vi "Find Album.vi"(8 "error in (no error)":errorcluster, 9 "Artist":string, 10 "Album":string, 11 "MusicLibrary in":refnum<class "MusicLibrary.lvclass">) -> (0 "error out":errorcluster, 2 "Album":refnum<class "Album.lvclass">, 3 "MusicLibrary out":refnum<class "MusicLibrary.lvclass">, 5 "Found?":bool)   [LabVIEW 2015, in "MusicLibrary.lvclass"]
uses:
  MusicLibrary.lvclass
  Album/Album.lvclass
  MusicElementLibrary.lvclass/MusicElementLibrary.ctl
  MusicElement.lvclass/MusicElement.ctl
  Album/Album.lvclass/Album.ctl
  MusicElement.lvclass
  MusicElementLibrary.lvclass
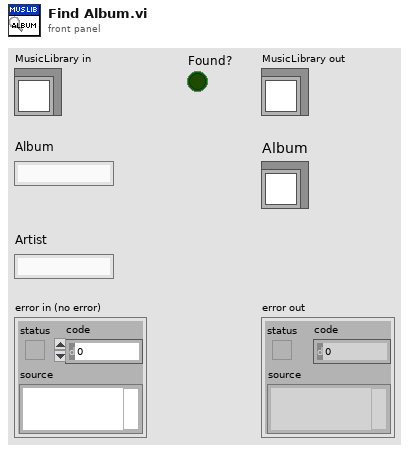
[diagram p1: front panel]
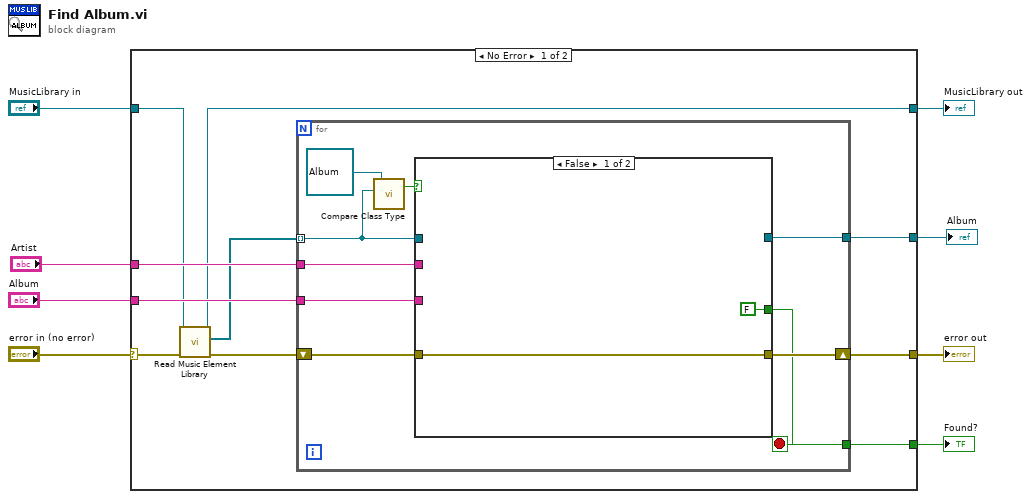
[diagram p0: block diagram]
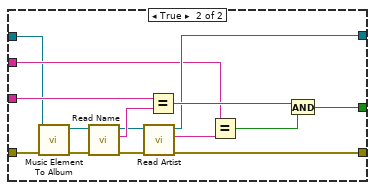
[diagram p2: hidden frame]
diagram:
  n1 = case shown="No Error" "error in (no error)" {
    selector: "error in (no error)" -> [w13 w46]
    tunnel: [w17 w46] -> w7
    tunnel: [w10 w45] -> w5
    tunnel: "MusicLibrary in" -> [w11 w45]
    tunnel: "Album" -> [w18 _]
    tunnel: [w15 _] -> w2
    tunnel: [w16 _] -> w3
    tunnel: "Artist" -> [w14 _]
    frame No Error {
      n2 = call "Read Music Element Library.vi"("error in (no error)"=w13, "MusicElementLibrary in"=w11) -> ("error out"=w12:errorcluster, "Music Element Library"=w9:refnum<class "MusicElement.lvclass">[], "MusicElementLibrary out"=w10:refnum<class "MusicLibrary.lvclass">)  [unwired: 7 in]
      n3 = for {
        tunnel: w9 -> [w19] mode=indexing
        shift-right: [w26] -> w17
        shift-left: w12 -> [w21]
        tunnel: w18 -> [w27]
        tunnel: [w25] -> w16
        tunnel: [w24] -> w15
        tunnel: w14 -> [w23]
        stop <- w25 stop-if-true
        n4 = call "Compare Class Type.vi"("MusicElement Check"=w19, "MusicElement in"=refnum<class "Album.lvclass"> refnum ("Album")) -> ("Same Class Type?"=w22:bool)  [unwired: 3 in]
        n5 = case shown="False" w22 {
          tunnel: w19 -> [_ w31]
          tunnel: w27 -> [_ w44]
          tunnel: [w29 w39] -> w26
          tunnel: [FALSE w41] -> w25
          tunnel: [_ w37] -> w24
          tunnel: w23 -> [_ w35]
          tunnel: w21 -> [w29 w33]
          frame False {
          }
          frame True {
            n6 = call "Music Element To Album.vi"("error in (no error)"=w33, "MusicElement"=w31) -> ("error out"=w32:errorcluster, "Album"=w30:refnum<class "Album.lvclass">)  [unwired: 8 in]
            n7 = call "Read Name.vi"("error in (no error)"=w32, "MusicElement in"=w30) -> ("error out"=w40:errorcluster, "Name"=w43:string, "MusicElement out"=w38:refnum<class "Album.lvclass">)  [unwired: 7 in]
            n8 = call "Read Artist.vi"("error in (no error)"=w40, "Album in"=w38) -> ("error out"=w39:errorcluster, "Artist"=w36:string, "Album out"=w37:refnum<class "Album.lvclass">)  [unwired: 7 in]
            n9 = Equal?(x=w44, y=w43) -> (x = y?=w42:bool)
            n10 = Equal?(x=w35, y=w36) -> (x = y?=w34:bool)
            n11 = And(x=w42, y=w34) -> (x .and. y?=w41:bool)
          }
        }
      }
    }
    frame Error {
    }
  }
  "error out" <- w7
  "MusicLibrary out" <- w5
  "Found?" <- w3
  "Album" <- w2
